vi "ziExample1-Module-DAQ_trigger.vi"() -> ()   [LabVIEW 2016]
doc: "Control a Zurich instrument device via the LabOne Labview API. \nRequirements: Zurich Instruments MFLI, HF2 or UHFLI \nThis example shows how to start a DAQ trigger module and retrieve the Data.\n\n© Zurich Instruments AG, www.zhinst.com"
uses:
  <instrlib>/Zurich Instruments LabOne/Public/Modules/ziTypeModEnum.ctl
  <instrlib>/Zurich Instruments LabOne/Public/Configure/ziSetValueDoubleArray.vi
  <instrlib>/Zurich Instruments LabOne/Public/Modules/ziModSetValueBinaryArray.vi
  <instrlib>/Zurich Instruments LabOne/Public/Modules/ziModSetValueDoubleArray.vi
  <instrlib>/Zurich Instruments LabOne/Public/Modules/ziModSetValueDouble.vi
  <instrlib>/Zurich Instruments LabOne/Public/Modules/ziModGetDoubleData.vi
  <instrlib>/Zurich Instruments LabOne/Zurich Instruments LabOne.lvlib
panel:
  in  "stop":bool
  in  "gridmode":bool
  out "Normal Demod R":dbl[][](graph)
  out "Grid DEMOD R":dbl[][](graph)
  out "Error Out":errorcluster
  in  "Address":string="DEV"
  out "Selected Device":string
  # "ziExample-Module-DAQ_trigger.vi\nRequirements: \n- HF2LI, UHFLI or MFLI \nsee block diagram for VI description"
  # "Tested Instruments:\n- HF2LI\n- UHFLI\n- MFLI"
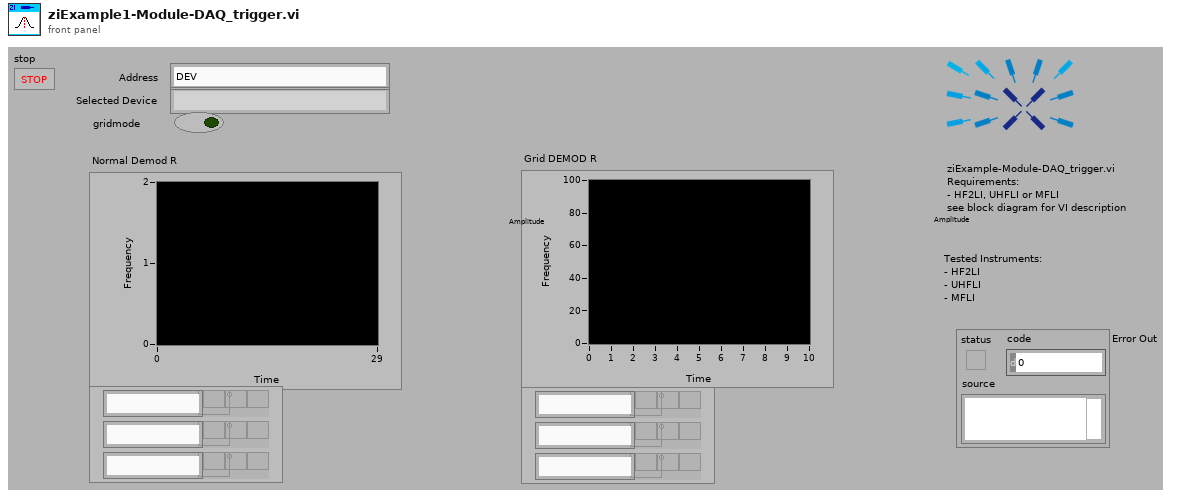
[diagram p1: front panel]
types:
  T1 = typedef "Zurich Instruments LabOne.lvlib/ziTypeModEnum.ctl" = u16
  T2 = typedef "Zurich Instruments LabOne.lvlib/ziTypeHandle.ctl" = cluster{"handleValid":bool, "Conn":u64, "Path Prefix":string, "Handle":u64, "Connected":bool, "Clockbase(s)":dbl}
  T3 = typedef "Zurich Instruments LabOne.lvlib/ziTypeModHandle.ctl" = cluster{"handleValid":bool, "Conn":u64, "ModHandle":u64, "moduleID":string, "Path Prefix":string}
  T4 = typedef "Zurich Instruments LabOne.lvlib/ziTypeModResults.ctl" = cluster{"PathArray":string[], "ValueType":T5, "NoOfResults":u64, "ziGenericHeader":T6[]}
  T5 = typedef "Zurich Instruments LabOne.lvlib/ziTypePollType.ctl" = enum16{"NONE", "DOUBLE_DATA", "INTEGER_DATA", "DEMOD_SAMPLE", "SCOPE_WAVE_HF2", "AUXIN_SAMPLE", "DIO_SAMPLE", "BYTE_ARRAY", "PWA_WAVE", "9", "10", "11", "12", "13", "14", "15", "TREE_CHANGE_DEPRI", "17", "ERROR", "19", "20", "21", "22", "23", "24", "25", "26", "27", "28", "29", "30", "31", "DOUBLE_DATA_TS", "INTEGER_DATA_TS", "34", "SCOPE_WAVE", "SCOPE_WAVE_EX", "37", "BYTE_ARRAY_TS", "39", "40", "41", "42", "43", "44", "45", "CNT_DATA", "47", "TREE_CHANGE", "49", "50", "51", "52", "53", "54", "55", "56", "57", "58", "59", "60", "61", "62", "63", "SWEEPER_DATA", "SPECTRUM_DATA", "ADVISOR_DATA", "VECTOR_DATA", "IMP_DATA"}
  T6 = typedef "Zurich Instruments LabOne.lvlib/ziTypeModGenericHeader.ctl" = cluster{"HeaderType":enum8{"HEADER_TYPE_NONE", "HEADER_TYPE_SWTRIGGER", "HEADER_TYPE_SWEEPER"}, "SampleFormat":u8, "SystemTime":timestamp, "CreatedTimeStamp":u64, "ChangedTimeStamp":u64, "Flags":u32, "ChunkSizeBytes":u64, "Name":string, "Status":u32, "GroupIndex":u32, "Color":u32, "ActiveRow":u32, "TriggerNumber":u64, "GridRows":u32, "GridCols":u32, "GridMode":u32, "GridOperation":u32, "GridDirection":u32, "GridRepetitions":u32, "GridColDelta":dbl, "GridColOffset":dbl, "GridRowDelta":dbl, "GridRowOffset":dbl, "Bandwidth":dbl, "Center":dbl, "Nenbw":dbl}
  T7 = typedef "Zurich Instruments LabOne.lvlib/ziTypeDoubleDataTSGrid.ctl" = cluster{"Timestamp (ticks)":u64[][], "Value":dbl[][]}
  T8 = typedef "Zurich Instruments LabOne.lvlib/ziTypeDoubleDataTS.ctl" = cluster{"Timestamp (ticks)":u64[], "Value":dbl[]}
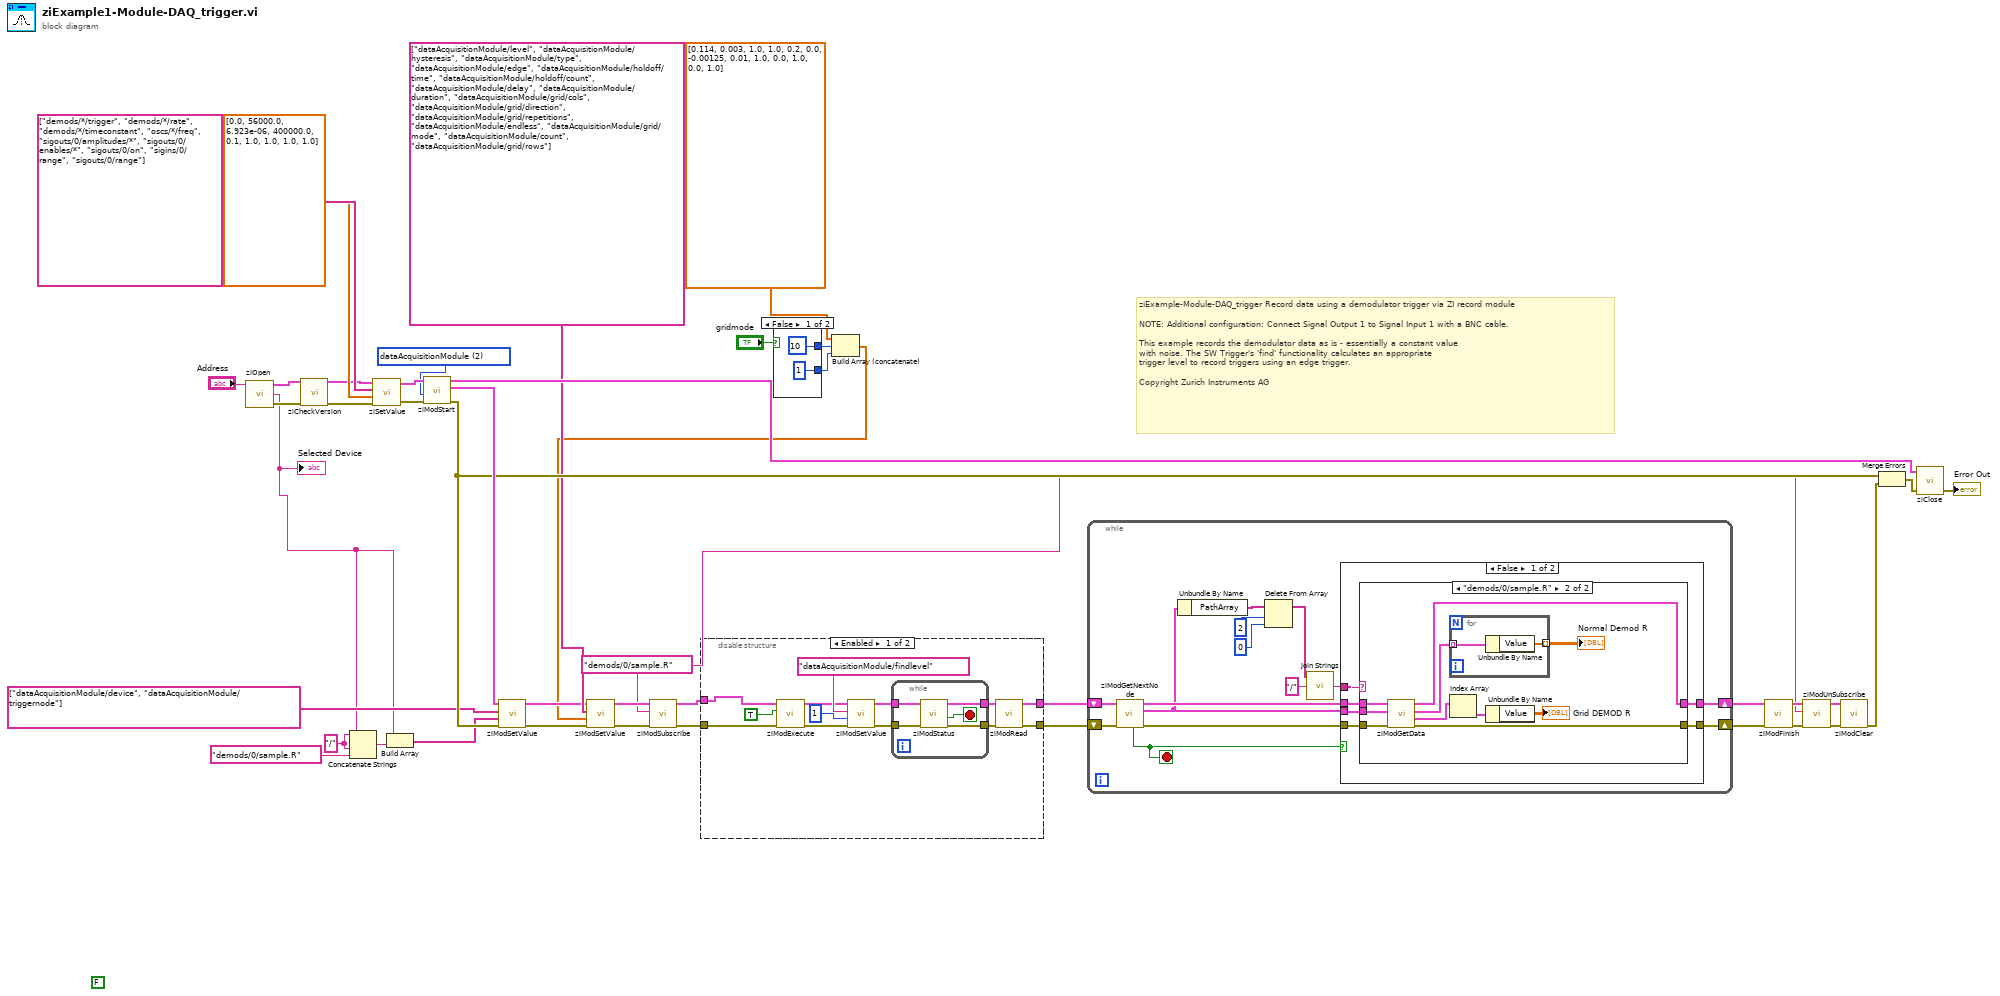
[diagram p0: block diagram]
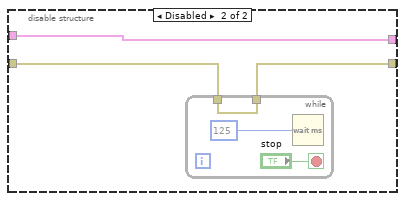
[diagram p2: hidden frame]
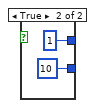
[diagram p3: hidden frame]
diagram:
  w5 = T1 2 items=["sweep", "scopeModule", "dataAcquisitionModule", "pidAdvisor", "awgModule", "impedanceModule", "multiDeviceSyncModule", "zoomFFT", "trigger", "deviceSettings", "record"] ("module Id")
  w14 = "/"
  w12 = "demods/0/sample.R" ("subscribe")
  (unwired) FALSE ("stop")
  # "ziExample-Module-DAQ_trigger Record data using a demodulator trigger via ZI record module\n \nNOTE: Additional configuration: Connect Signal Output 1 to Signal Input 1 with a BNC cable.\n\nThis example records the demodulator data as is - essentially a constant value\nwith noise. The SW Trigger's 'find' functionality calculates an appropriate\ntrigger level to record triggers using an edge trigger.\n\nCopyright Zurich Instruments AG"
  n1 = call <instrlib>:"ziOpen.vi"("Address"="Address") -> ("Error Out"=w27:errorcluster, "Selected Device"=w13:string, "HandleOut"=w30:T2)  [unwired: 1 in, 2 out]
  "Selected Device" <- w13
  n2 = call <instrlib>:"ziCheckVersion.vi"("Handle In"=w30, "Error In"=w27) -> ("Handle Out"=w29:T2, "Error Out"=w28:errorcluster)  [unwired: 11 in, 1 out]
  n3 = Concatenate Strings(w14, w13, w14, "demods/0/sample.R" ("element")) -> (w11:string)
  n4 = call-poly <instrlib>:"ziSetValue.vi"("Error In"=w28, "Values"=dbl[] [0.0, 56000.0, 6.923e-06, 400000.0, 0.1, 1.0, 1.0, 1.0, 1.0], "Paths"=string[] ["demods/*/trigger", "demods/*/rate", "demods/*/timeconstant", "oscs/*/freq", "sigouts/0/amplitudes/*", "sigouts/0/enables/*", "sigouts/0/on", "sigins/0/range", "sigouts/0/range"], "Handle In"=w29) -> ("Error Out"=w37:errorcluster, "Handle Out"=w36:T2)  [unwired: 1 in]
  n5 = Build Array(w13, w11) -> (w21:string[])
  n6 = call <instrlib>:"ziModStart.vi"("Error In"=w37, "module Id"=w5, "Handle In"=w36) -> ("Error Out"=w32:errorcluster, "ModHandle Out"=w35:T3, "Handle Out"=w31:T2)  [unwired: 6 in]
  n7 = call-poly <instrlib>:"ziModSetValue.vi"("Error In"=w32, "Values"=w21, "Paths"=string[] ["dataAcquisitionModule/device", "dataAcquisitionModule/triggernode"], "ModHandle In"=w35) -> ("Error Out"=w18:errorcluster, "ModHandle Out"=w19:T3)  [unwired: 6 in]
  n8 = case shown="False" "gridmode" {
    tunnel: [10 1] -> w8
    tunnel: [1 10] -> w7
    frame False {
    }
    frame True {
    }
  }
  n9 = Build Array (concatenate)(dbl[] [0.114, 0.003, 1.0, 1.0, 0.2, 0.0, -0.00125, 0.01, 1.0, 0.0, 1.0, 0.0, 1.0], w8, w7) -> (w6:dbl[])
  n10 = call-poly <instrlib>:"ziModSetValue.vi"("Error In"=w18, "Values"=w6, "Paths"=string[] ["dataAcquisitionModule/level", "dataAcquisitionModule/hysteresis", "dataAcquisitionModule/type", "dataAcquisitionModule/edge", "dataAcquisitionModule/holdoff/time", "dataAcquisitionModule/holdoff/count", "dataAcquisitionModule/delay", "dataAcquisitionModule/duration", "dataAcquisitionModule/grid/cols", "dataAcquisitionModule/grid/direction", "dataAcquisitionModule/grid/repetitions", "dataAcquisitionModule/endless", "dataAcquisitionModule/grid/mode", "dataAcquisitionModule/count", "dataAcquisitionModule/grid/rows"], "ModHandle In"=w19) -> ("Error Out"=w16:errorcluster, "ModHandle Out"=w17:T3)  [unwired: 6 in]
  n11 = call <instrlib>:"ziModSubscribe.vi"("Error In"=w16, "Path"=w12, "ModHandle In"=w17) -> ("Error Out"=w1:errorcluster, "ModHandle Out"=w2:T3)  [unwired: 6 in]
  n12 = disable-structure shown="Enabled" {
    disable-tunnel: w2 -> [w55 w68]
    disable-tunnel: w1 -> [w52 w67]
    disable-tunnel: [w48 w68] -> w4
    disable-tunnel: [w50 w66] -> w3
    frame Enabled {
      n13 = call <instrlib>:"ziModExecute.vi"("Error In"=w52, "Modal (F)"=TRUE, "ziModHandle In"=w55) -> ("Error Out"=w54:errorcluster, "ziModHandle Out"=w53:T3)  [unwired: 5 in, 1 out]
      n14 = call-poly <instrlib>:"ziModSetValue.vi"("Error In"=w54, "Value"=1, "Path"="dataAcquisitionModule/findlevel", "ModHandle In"=w53) -> ("Error Out"=w58:errorcluster, "ModHandle Out"=w59:T3)  [unwired: 6 in]
      n15 = while {
        tunnel: w59 -> [w65]
        tunnel: w58 -> [w64]
        tunnel: [w62] -> w49
        tunnel: [w61] -> w51
        stop <- w63 stop-if-true
        n16 = call <instrlib>:"ziModStatus.vi"("Error In"=w64, "ModHandle IN"=w65) -> ("Error Out"=w61:errorcluster, "Finished?"=w63:bool, "ModHandle Out"=w62:T3)  [unwired: 5 in, 1 out]
      }
      n17 = call <instrlib>:"ziModRead.vi"("error in"=w51, "ziModHandle In"=w49) -> ("error out"=w50:errorcluster, "ziModHandle Out"=w48:T3)  [unwired: 8 in]
    }
    frame Disabled {
      n18 = while {
        tunnel: w67 -> [w69]
        tunnel: [w69] -> w66
        stop <- "stop" stop-if-true
        n19 = Wait (ms)(milliseconds to wait=u32 125) -> ()  [unwired: 1 out]
      }
    }
  }
  n20 = while {
    shift-right: [w80] -> w24
    shift-left: w4 -> [w84]
    shift-right: [w81] -> w25
    shift-left: w3 -> [w85]
    stop <- w79 stop-if-true
    n21 = call <instrlib>:"ziModGetNextNode.vi"("Error In"=w85, "ModHandle In"=w84) -> ("Error Out"=w82:errorcluster, "ModResults"=w78:T4, "ModHandle Out"=w83:T3, "NoData"=w79:bool)  [unwired: 6 in]
    n22 = Unbundle By Name(w78) -> ("PathArray"=w77:string[])
    n23 = Delete From Array(array=w77, length=2, index=0) -> (array with subset deleted=w74:string[])  [unwired: 1 out]
    n24 = call <vilib>:"Join Strings.vi"("Separator (,)"="/", "Strings In"=w74) -> ("String"=w72:string)  [unwired: 1 in]
    n25 = case shown="False" w79 {
      tunnel: w78 -> [w91 _]
      tunnel: w83 -> [w90 w107]
      tunnel: w82 -> [w89 w106]
      tunnel: [w88 w106] -> w81
      tunnel: [w87 w107] -> w80
      tunnel: w72 -> [w86 _]
      frame False {
        n26 = case shown="\"demods/0/sample.R\"" w86 {
          tunnel: w90 -> [w93 w97]
          tunnel: w91 -> [_ w96]
          tunnel: w89 -> [w92 w100]
          tunnel: [w92 w102] -> w88
          tunnel: [w93 w103] -> w87
          frame Default {
          }
          frame "demods/0/sample.R" {
            n27 = call-poly <instrlib>:"ziModGetData.vi"("Error In"=w100, "ModResults"=w96, "ModHandle In"=w97) -> ("Error Out"=w102:errorcluster, "DoubleSampleGrid"=w99:T7[], "DoubleSample"=w101:T8[], "ModHandle Out"=w103:T3)  [unwired: 4 in, 1 out]
            n28 = for {
              tunnel: w101 -> [w105] mode=indexing
              tunnel: [w104] -> w94 mode=indexing
              n29 = Unbundle By Name(w105) -> ("Value"=w104:dbl[])
            }
            "Normal Demod R" <- w94
            n30 = Index Array(array=w99) -> (element=w98:T7)  [unwired: 1 in]
            n31 = Unbundle By Name(w98) -> ("Value"=→"Grid DEMOD R":dbl[][])
          }
        }
      }
      frame True {
      }
    }
  }
  n32 = call <instrlib>:"ziModFinish.vi"("Error In"=w25, "ziModHandle In"=w24) -> ("Error Out"=w26:errorcluster, "ziModHandle Out"=w23:T3)  [unwired: 7 in]
  n33 = call <instrlib>:"ziModUnSubscribe.vi"("Error In"=w26, "Path (\"/\")"=w12, "ModHandle In"=w23) -> ("Error Out"=w42:errorcluster, "ModHandle Out"=w41:T3)  [unwired: 7 in]
  n34 = call <instrlib>:"ziModClear.vi"("Error In"=w42, "ziModHandle In"=w41) -> ("Error Out"=w34:errorcluster)  [unwired: 7 in, 1 out]
  n35 = Merge Errors(w32, w34) -> (w33:errorcluster)
  n36 = call <instrlib>:"ziClose.vi"("Error In"=w33, "Handle In"=w31) -> ("Error Out"=→"Error Out":errorcluster)  [unwired: 2 in, 1 out]
